vi "Rotation2d_Interpolate.vi"(9 "T":dbl, 10 "EncValue ROTATION":T1={"VALUE"=0.0, "COS"=1.0, "SIN"=0.0} {"SIN" format="%13.4f"; "COS" format="%13.4f"; "VALUE" format="%13.4f"}, 11 "in ROTATION":T1={"VALUE"=0.0, "COS"=1.0, "SIN"=0.0} {"SIN" format="%13.4f"; "COS" format="%13.4f"; "VALUE" format="%13.4f"}) -> (3 "Interpolated ROTATION":T1 {"SIN" format="%13.4f"; "COS" format="%13.4f"; "VALUE" format="%13.4f"})   [LabVIEW 2019, in "Trajectory_Library.lvlib"]
doc: "Interpolate between 2 rotations\n\nParameters:\n- in ROTATION - This rotation data structure\n - EndValue ROTATION - The end value rotation\n - T -- Value between 0 and 1.\n\nReturns:\n - Interpolated ROTATION - The interpolated rotation."
uses:
  Trajectory_Library.lvlib
  TypeDef/ROTATION2D.ctl
  Rotation2d_RotateBy.vi
  Rotation2d_UnaryMinus.vi
  Rotation2d_CreateAngle.vi
  Rotation2d_CreateXY.vi
  Util_CalcDist.vi
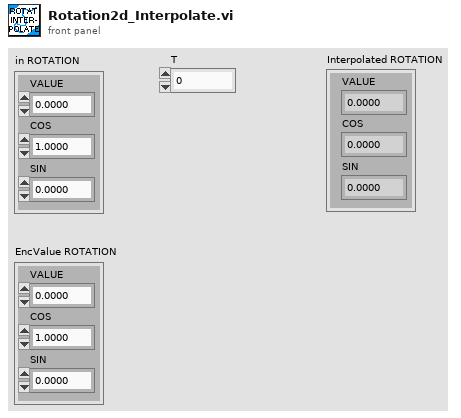
[diagram p1: front panel]
types:
  T1 = typedef "Trajectory_Library.lvlib/ROTATION2D.ctl" = cluster{"VALUE":dbl, "COS":dbl, "SIN":dbl}
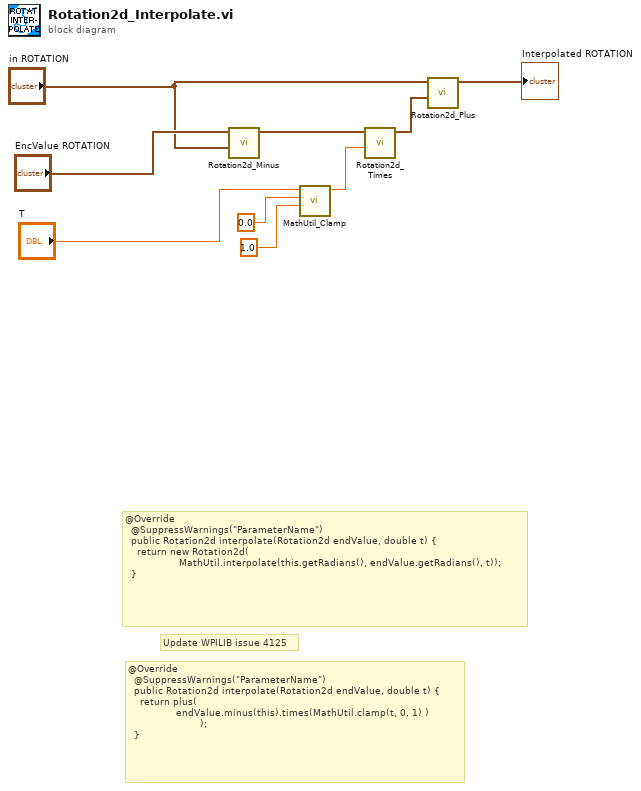
[diagram p0: block diagram]
diagram:
  # "Update WPILIB issue 4125"
  # "@Override\n  @SuppressWarnings(\"ParameterName\")\n  public Rotation2d interpolate(Rotation2d endValue, double t) {\n    return plus(\n                endValue.minus(this).times(MathUtil.clamp(t, 0, 1) ) \n                        );\n  }"
  # "@Override\n  @SuppressWarnings(\"ParameterName\")\n  public Rotation2d interpolate(Rotation2d endValue, double t) {\n    return new Rotation2d(\n                  MathUtil.interpolate(this.getRadians(), endValue.getRadians(), t));\n  }"
  n1 = call "Rotation2d_Minus.vi"("other ROTATION"="in ROTATION", "in ROTATION"="EncValue ROTATION") -> ("out ROTATION"=w4:T1)  [unwired: 9 in]
  n2 = call "MathUtil_Clamp.vi"("High Limit"=1.0, "Low Limit"=0.0, "Value"="T") -> ("Result"=w3:dbl)  [unwired: 8 in]
  n3 = call "Rotation2d_Times.vi"("Scalar"=w3, "in ROTATION"=w4) -> ("out ROTATION"=w2:T1)  [unwired: 9 in]
  n4 = call "Rotation2d_Plus.vi"("other ROTATION"=w2, "in ROTATION"="in ROTATION") -> ("out ROTATION"=→"Interpolated ROTATION":T1)  [unwired: 9 in]
